vi "Create All Message Queues.vi"(8 "error in (no error)":errorcluster) -> (0 "error out":errorcluster, 3 "Message Queues out":T1)   [LabVIEW 2020, in "Message Queue.lvlib"]
doc: "This VI creates and initializes all the message queues for your application. If your application requires more than one message queue, right-click the \"Message Queues\" constant above and select Open Type Def. Add the new Message Queue(s) to the type definition, then initialize them in this VI."
uses:
  Message Queue.lvlib
  All Message Queues.ctl
  Message Cluster.ctl
  Enqueue Message (Single).vi
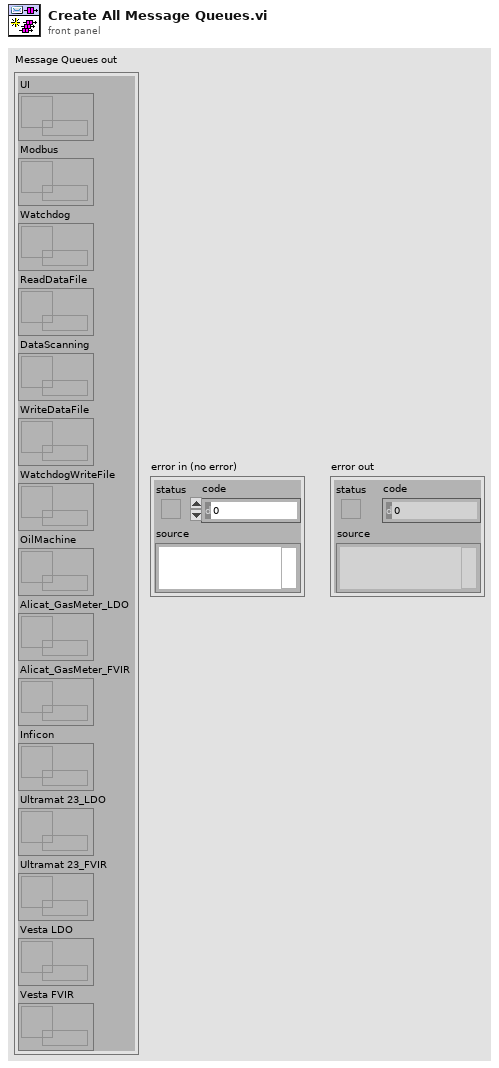
[diagram p1: front panel]
types:
  T1 = typedef "Message Queue.lvlib/All Message Queues.ctl" = cluster{"UI":refnum<queue>, "Modbus":refnum<queue>, "Watchdog":refnum<queue>, "ReadDataFile":refnum<queue>, "DataScanning":refnum<queue>, "WriteDataFile":refnum<queue>, "WatchdogWriteFile":refnum<queue>, "OilMachine":refnum<queue>, "Alicat_GasMeter_LDO":refnum<queue>, "Inficon":refnum<queue>, "Ultramat 23_LDO":refnum<queue>, "Alicat_GasMeter_FVIR":refnum<queue>, "Ultramat 23_FVIR":refnum<queue>, "Vesta LDO":refnum<queue>, "Vesta FVIR":refnum<queue>}
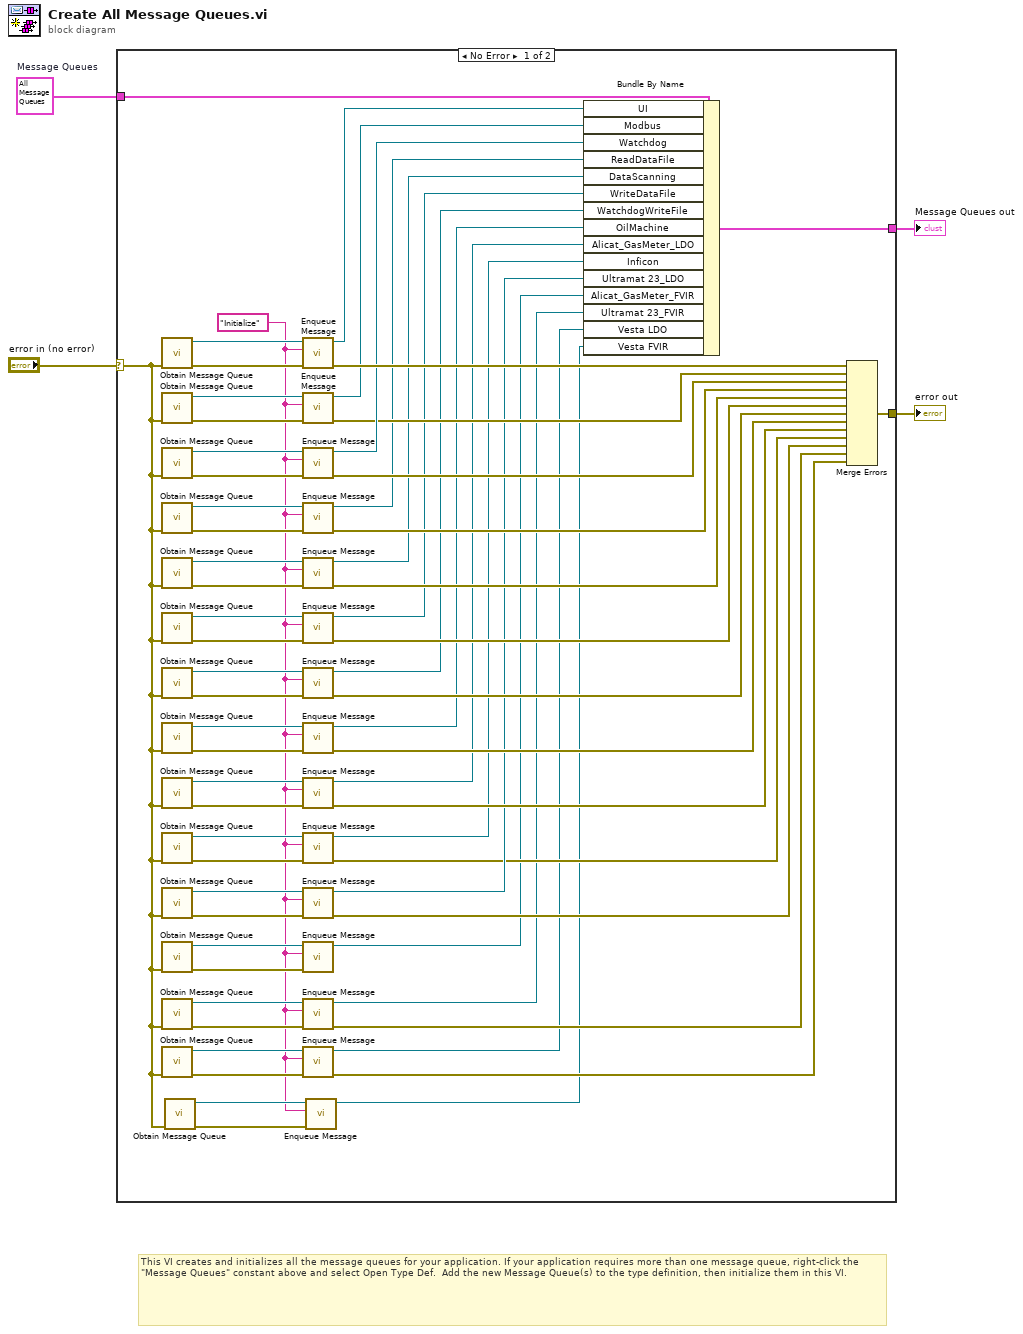
[diagram p0: block diagram]
diagram:
  w1 = T1 {"UI"=refnum, "Modbus"=refnum, "Watchdog"=refnum, "ReadDataFile"=refnum, "DataScanning"=refnum, "WriteDataFile"=refnum, "WatchdogWriteFile"=refnum, "OilMachine"=refnum, "Alicat_GasMeter_LDO"=refnum, "Inficon"=refnum, "Ultramat 23_LDO"=refnum, "Alicat_GasMeter_FVIR"=refnum, "Ultramat 23_FVIR"=refnum, "Vesta LDO"=refnum, "Vesta FVIR"=refnum}  # Message Queues
  # "This VI creates and initializes all the message queues for your application. If your application requires more than one message queue, right-click the \"Message Queues\" constant above and select Open Type Def.  Add the new Message Queue(s) to the type definition, then initialize them in this VI."
  n1 = case shown="No Error" "error in (no error)" {
    selector: "error in (no error)" -> [w7 w69]
    tunnel: [w47 w69] -> w4
    tunnel: [w66 w68] -> w2
    tunnel: w1 -> [w14 w68]
    frame No Error {
      w6 = "Initialize" ("Message")
      n2 = call "Obtain Message Queue.vi"("error in (no error)"=w7) -> ("error out"=w65:errorcluster, "Message Queue"=w64:refnum<queue>)  [unwired: 9 in]
      n3 = call "Obtain Message Queue.vi"("error in (no error)"=w7) -> ("error out"=w62:errorcluster, "Message Queue"=w63:refnum<queue>)  [unwired: 9 in]
      n4 = call "Obtain Message Queue.vi"("error in (no error)"=w7) -> ("error out"=w61:errorcluster, "Message Queue"=w60:refnum<queue>)  [unwired: 9 in]
      n5 = call "Obtain Message Queue.vi"("error in (no error)"=w7) -> ("error out"=w54:errorcluster, "Message Queue"=w53:refnum<queue>)  [unwired: 9 in]
      n6 = call "Obtain Message Queue.vi"("error in (no error)"=w7) -> ("error out"=w50:errorcluster, "Message Queue"=w49:refnum<queue>)  [unwired: 9 in]
      n7 = call "Obtain Message Queue.vi"("error in (no error)"=w7) -> ("error out"=w45:errorcluster, "Message Queue"=w43:refnum<queue>)  [unwired: 9 in]
      n8 = call "Obtain Message Queue.vi"("error in (no error)"=w7) -> ("error out"=w41:errorcluster, "Message Queue"=w38:refnum<queue>)  [unwired: 9 in]
      n9 = call "Obtain Message Queue.vi"("error in (no error)"=w7) -> ("error out"=w37:errorcluster, "Message Queue"=w34:refnum<queue>)  [unwired: 9 in]
      n10 = call "Obtain Message Queue.vi"("error in (no error)"=w7) -> ("error out"=w32:errorcluster, "Message Queue"=w33:refnum<queue>)  [unwired: 9 in]
      n11 = call "Obtain Message Queue.vi"("error in (no error)"=w7) -> ("error out"=w29:errorcluster, "Message Queue"=w28:refnum<queue>)  [unwired: 9 in]
      n12 = call "Obtain Message Queue.vi"("error in (no error)"=w7) -> ("error out"=w25:errorcluster, "Message Queue"=w26:refnum<queue>)  [unwired: 9 in]
      n13 = call "Obtain Message Queue.vi"("error in (no error)"=w7) -> ("error out"=w21:errorcluster, "Message Queue"=w20:refnum<queue>)  [unwired: 9 in]
      n14 = call "Obtain Message Queue.vi"("error in (no error)"=w7) -> ("error out"=w18:errorcluster, "Message Queue"=w17:refnum<queue>)  [unwired: 9 in]
      n15 = call "Obtain Message Queue.vi"("error in (no error)"=w7) -> ("error out"=w13:errorcluster, "Message Queue"=w12:refnum<queue>)  [unwired: 9 in]
      n16 = call "Obtain Message Queue.vi"("error in (no error)"=w7) -> ("error out"=w8:errorcluster, "Message Queue"=w9:refnum<queue>)  [unwired: 9 in]
      n17 = call-poly "Enqueue Message.vi"("error in (no error)"=w65, "Message"=w6, "Message Queue"=w64) -> ("error out"=w67:errorcluster, "dup Message Queue"=w59:refnum<queue>)  [unwired: 7 in]
      n18 = call-poly "Enqueue Message.vi"("error in (no error)"=w62, "Message"=w6, "Message Queue"=w63) -> ("error out"=w56:errorcluster, "dup Message Queue"=w58:refnum<queue>)  [unwired: 7 in]
      n19 = call-poly "Enqueue Message.vi"("error in (no error)"=w61, "Message"=w6, "Message Queue"=w60) -> ("error out"=w55:errorcluster, "dup Message Queue"=w57:refnum<queue>)  [unwired: 7 in]
      n20 = call-poly "Enqueue Message.vi"("error in (no error)"=w54, "Message"=w6, "Message Queue"=w53) -> ("error out"=w52:errorcluster, "dup Message Queue"=w51:refnum<queue>)  [unwired: 7 in]
      n21 = call-poly "Enqueue Message.vi"("error in (no error)"=w50, "Message"=w6, "Message Queue"=w49) -> ("error out"=w48:errorcluster, "dup Message Queue"=w46:refnum<queue>)  [unwired: 7 in]
      n22 = call-poly "Enqueue Message.vi"("error in (no error)"=w45, "Message"=w6, "Message Queue"=w43) -> ("error out"=w42:errorcluster, "dup Message Queue"=w44:refnum<queue>)  [unwired: 7 in]
      n23 = call-poly "Enqueue Message.vi"("error in (no error)"=w41, "Message"=w6, "Message Queue"=w38) -> ("error out"=w40:errorcluster, "dup Message Queue"=w39:refnum<queue>)  [unwired: 7 in]
      n24 = call-poly "Enqueue Message.vi"("error in (no error)"=w37, "Message"=w6, "Message Queue"=w34) -> ("error out"=w36:errorcluster, "dup Message Queue"=w35:refnum<queue>)  [unwired: 7 in]
      n25 = call-poly "Enqueue Message.vi"("error in (no error)"=w32, "Message"=w6, "Message Queue"=w33) -> ("error out"=w31:errorcluster, "dup Message Queue"=w30:refnum<queue>)  [unwired: 7 in]
      n26 = call-poly "Enqueue Message.vi"("error in (no error)"=w29, "Message"=w6, "Message Queue"=w28) -> ("error out"=w23:errorcluster, "dup Message Queue"=w27:refnum<queue>)  [unwired: 7 in]
      n27 = call-poly "Enqueue Message.vi"("error in (no error)"=w25, "Message"=w6, "Message Queue"=w26) -> ("error out"=w22:errorcluster, "dup Message Queue"=w24:refnum<queue>)  [unwired: 7 in]
      n28 = call-poly "Enqueue Message.vi"("error in (no error)"=w21, "Message"=w6, "Message Queue"=w20) -> ("dup Message Queue"=w19:refnum<queue>)  [unwired: 7 in, 1 out]
      n29 = call-poly "Enqueue Message.vi"("error in (no error)"=w18, "Message"=w6, "Message Queue"=w17) -> ("error out"=w15:errorcluster, "dup Message Queue"=w16:refnum<queue>)  [unwired: 7 in]
      n30 = call-poly "Enqueue Message.vi"("error in (no error)"=w13, "Message"=w6, "Message Queue"=w12) -> ("error out"=w11:errorcluster, "dup Message Queue"=w10:refnum<queue>)  [unwired: 7 in]
      n31 = call-poly "Enqueue Message.vi"("error in (no error)"=w8, "Message"=w6, "Message Queue"=w9) -> ("dup Message Queue"=w5:refnum<queue>)  [unwired: 7 in, 1 out]
      n32 = Bundle By Name(cluster=w14, "UI"=w59, "Modbus"=w58, "Watchdog"=w57, "ReadDataFile"=w51, "DataScanning"=w46, "WriteDataFile"=w44, "WatchdogWriteFile"=w39, "OilMachine"=w35, "Alicat_GasMeter_LDO"=w30, "Inficon"=w27, "Ultramat 23_LDO"=w24, "Alicat_GasMeter_FVIR"=w19, "Ultramat 23_FVIR"=w16, "Vesta LDO"=w10, "Vesta FVIR"=w5) -> (w66:T1)
      n33 = Merge Errors(w67, w56, w55, w52, w48, w42, w40, w36, w31, w23, w22, w15, w11) -> (w47:errorcluster)
    }
    frame Error {
    }
  }
  "Message Queues out" <- w2
  "error out" <- w4
